vi "Force Mirror.vi"(8 "error in":errorcluster, 11 "CR5 in":refnum<class "CR5.lvclass">) -> (0 "error out":errorcluster, 3 "CR5 out":refnum<class "CR5.lvclass">)   [LabVIEW 2015, in "CR5.lvclass"]
doc: "Force mirror to -40degC."
uses:
  CR5.lvclass
  Reusable/Session APIs/Serial/Serial Session.lvclass
  CR5.lvclass/CR5.ctl
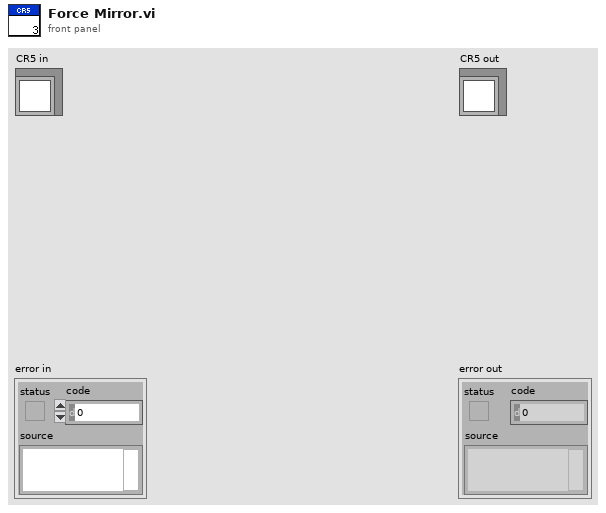
[diagram p1: front panel]
types:
  T1 = typedef "Session - Root.lvclass/Session Handle.ctl" = refnum<data-value>
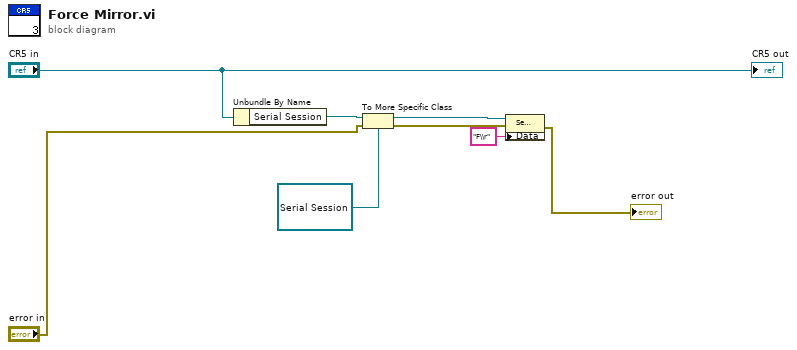
[diagram p0: block diagram]
diagram:
  n1 = Unbundle By Name("CR5 in") -> ("Serial Session"=w7:T1)
  n2 = To More Specific Class(target class=refnum<data-value> refnum, reference=w7, error in="error in") -> (specific class reference=w3:refnum<data-value>, error out=w4:errorcluster)
  n3 = property class="Serial Session"(reference=w3, error in=w4, "Data"="F\\r") -> (error out=→"error out":errorcluster)  [unwired: 1 out]
  "CR5 out" <- "CR5 in"
